vi "Get Motor Velocity Setpoint.vi"(8 "error in (no error)":errorcluster, 11 "wheel in":refnum<class "NI_Robotics_Wheel.lvclass">) -> (0 "error out":errorcluster, 1 "failed?":bool, 2 "ccw motor velocity setpoint":dbl, 3 "wheel out":refnum<class "NI_Robotics_Wheel.lvclass">)   [LabVIEW 2017, in "NI_Robotics_Wheel.lvclass"]
uses:
  <vilib>/robotics/Steering/Wheel/NI_Robotics_Wheel.lvclass
  <vilib>/robotics/Steering/Wheel/NI_Robotics_Wheel.lvclass/NI_Robotics_Wheel.ctl
  <vilib>/robotics/Actuation/Motor Communication/NI_Robotics_Motor Communication.lvclass
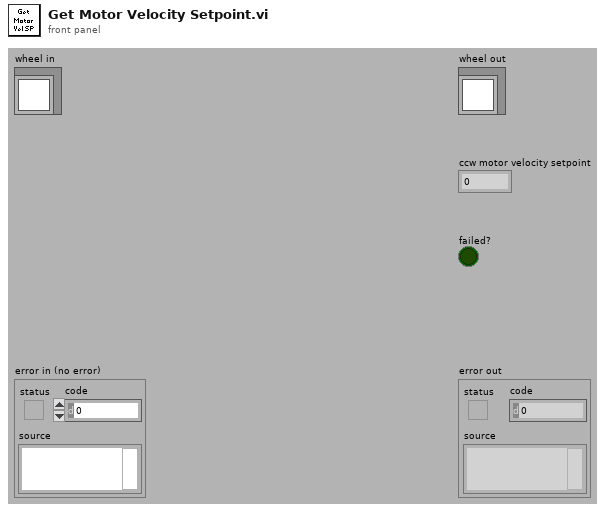
[diagram p1: front panel]
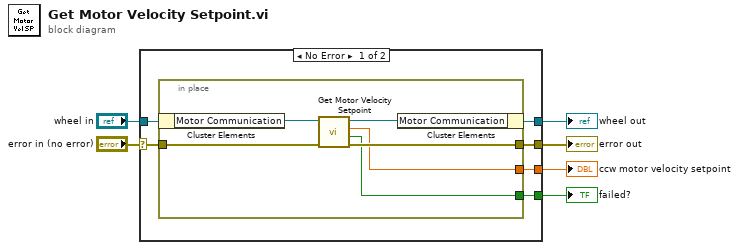
[diagram p0: block diagram]
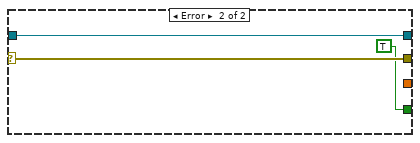
[diagram p2: hidden frame]
diagram:
  n1 = case shown="No Error" "error in (no error)" {
    selector: "error in (no error)" -> [w10 w21]
    tunnel: [w9 w21] -> w5
    tunnel: [w11 w20] -> w3
    tunnel: "wheel in" -> [w12 w20]
    tunnel: [w8 _] -> w2
    tunnel: [w7 TRUE ("failed?")] -> w1
    frame No Error {
      n2 = in-place {
        in-place-border: [w16] -> w9
        in-place-border: w10 -> [w15]
        in-place-border: [w14] -> w8
        in-place-border: [w13] -> w7
        n3 = in-place-cluster #1(w12) -> ("Motor Communication"=w18:refnum<class "NI_Robotics_Motor Communication.lvclass">)
        n4 = call <vilib>:"Get Motor Velocity Setpoint.vi"("error in (no error)"=w15, "motor communication in"=w18) -> ("error out"=w16:errorcluster, "failed?"=w13:bool, "velocity"=w14:dbl, "motor communication out"=w17:refnum<class "NI_Robotics_Motor Communication.lvclass">)  [unwired: 6 in]
        n5 = in-place-cluster #1("Motor Communication"=w17) -> (w11:refnum<class "NI_Robotics_Wheel.lvclass">)
      }
    }
    frame Error {
    }
  }
  "error out" <- w5
  "wheel out" <- w3
  "ccw motor velocity setpoint" <- w2
  "failed?" <- w1
